vi "MH_ChSumm.vi"(11 "HistDat":cluster{dbl, dbl, dbl, dbl}[](array[cluster])) -> (3 "HistDat Out":cluster{dbl, dbl, dbl, dbl}[](array[cluster]))   [LabVIEW 2019]
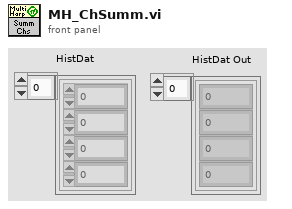
[diagram p1: front panel]
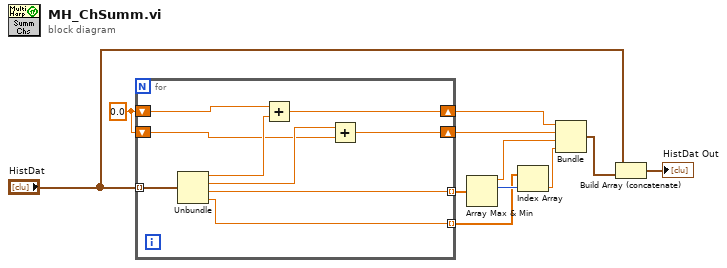
[diagram p0: block diagram]
diagram:
  w10 = 0.0
  n1 = for {
    tunnel: "HistDat" -> [w20] mode=indexing
    shift-right: [w17] -> w9
    shift-left: w10 -> [w19]
    tunnel: [w16] -> w11 mode=indexing
    tunnel: [w15] -> w5 mode=indexing
    shift-right: [w13] -> w8
    shift-left: w10 -> [w12]
    n2 = Unbundle(w20) -> (w18:dbl, w14:dbl, w16:dbl, w15:dbl)
    n3 = Add(x=w19, y=w18) -> (x+y=w17:dbl)
    n4 = Add(x=w14, y=w12) -> (x+y=w13:dbl)
  }
  n5 = Array Max & Min(array=w11) -> (max value=w7:dbl, max index (indices)=w6:i32)  [unwired: 2 out]
  n6 = Index Array(array=w5, index=w6) -> (element=w4:dbl)
  n7 = Bundle(w9, w8, w7, w4) -> (w2:cluster{dbl, dbl, dbl, dbl})  [unwired: 1 in]
  n8 = Build Array (concatenate)("HistDat", w2) -> (→"HistDat Out":cluster{dbl, dbl, dbl, dbl}[])
